vi "ExecutingCalibration.vi"(8 "error in (no error)":errorcluster, 10 "calibration_id":i32, 11 "ByteGSAPIBase in":refnum<class "ByteQXAPIBase.lvclass">) -> (0 "error out":errorcluster, 2 "calibration data":T1 {"controls"."umidita" format="%.1g"; "controls"."temperatura_c" format="%.1g"; "controls"."incertezza" format="%.1g"; "controls"."deviazione_standard" format="%.1g"; "controls"."mpe_min" format="%.1g"; "controls"."mpe_max" format="%.1g"; "controls"."riferimento_obiettivo" format="%.1g"}, 3 "ByteGSAPIBase out":refnum<class "ByteQXAPIBase.lvclass">)   [LabVIEW 2019, in "ByteQXWebAPI.lvlib" / "ByteQXAPIBase.lvclass"]
doc: "Obtain calibration measurements for the specified calibration Id"
uses:
  ByteQXAPIBase.lvclass
  BodyCalibrazioneMisure.ctl
  <vilib>/Bytelabs/ByteREST/ByteRESTClass/ByteRESTBase/HTTP/Status_Code.ctl
  ByteQXAPIBase.lvclass/ByteQXAPIBase.ctl
  <vilib>/Utility/error.llb/Error Cluster From Error Code.vi
  <vilib>/ErrorRing/Error Ring.xnode
  <vilib>/Bytelabs/ByteREST/ByteRESTClass/ByteRESTBase/RESTBase.lvclass
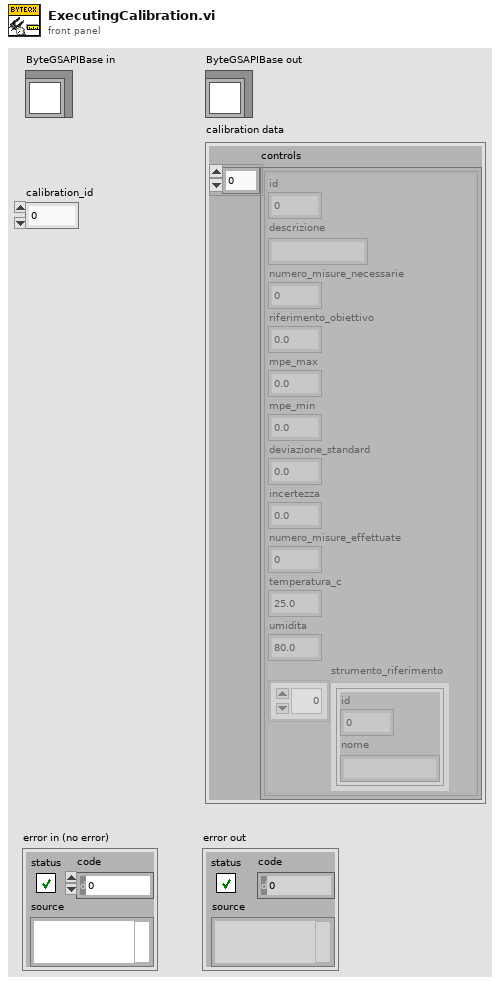
[diagram p1: front panel]
types:
  T1 = typedef "ByteQXWebAPI.lvlib/ByteQXAPIBase.lvclass/BodyCalibrazioneMisure.ctl" = cluster{"controls":cluster{"id":u16, "descrizione":string, "numero_misure_necessarie":u16, "riferimento_obiettivo":dbl, "mpe_max":dbl, "mpe_min":dbl, "deviazione_standard":dbl, "incertezza":dbl, "numero_misure_effettuate":u32, "temperatura_c":dbl, "umidita":dbl, "strumento_riferimento":cluster{"id":u16, "nome":string}[]}[]}
  T2 = typedef "ByteREST.lvlib/RESTBase.lvclass/Status_Code.ctl" = u16
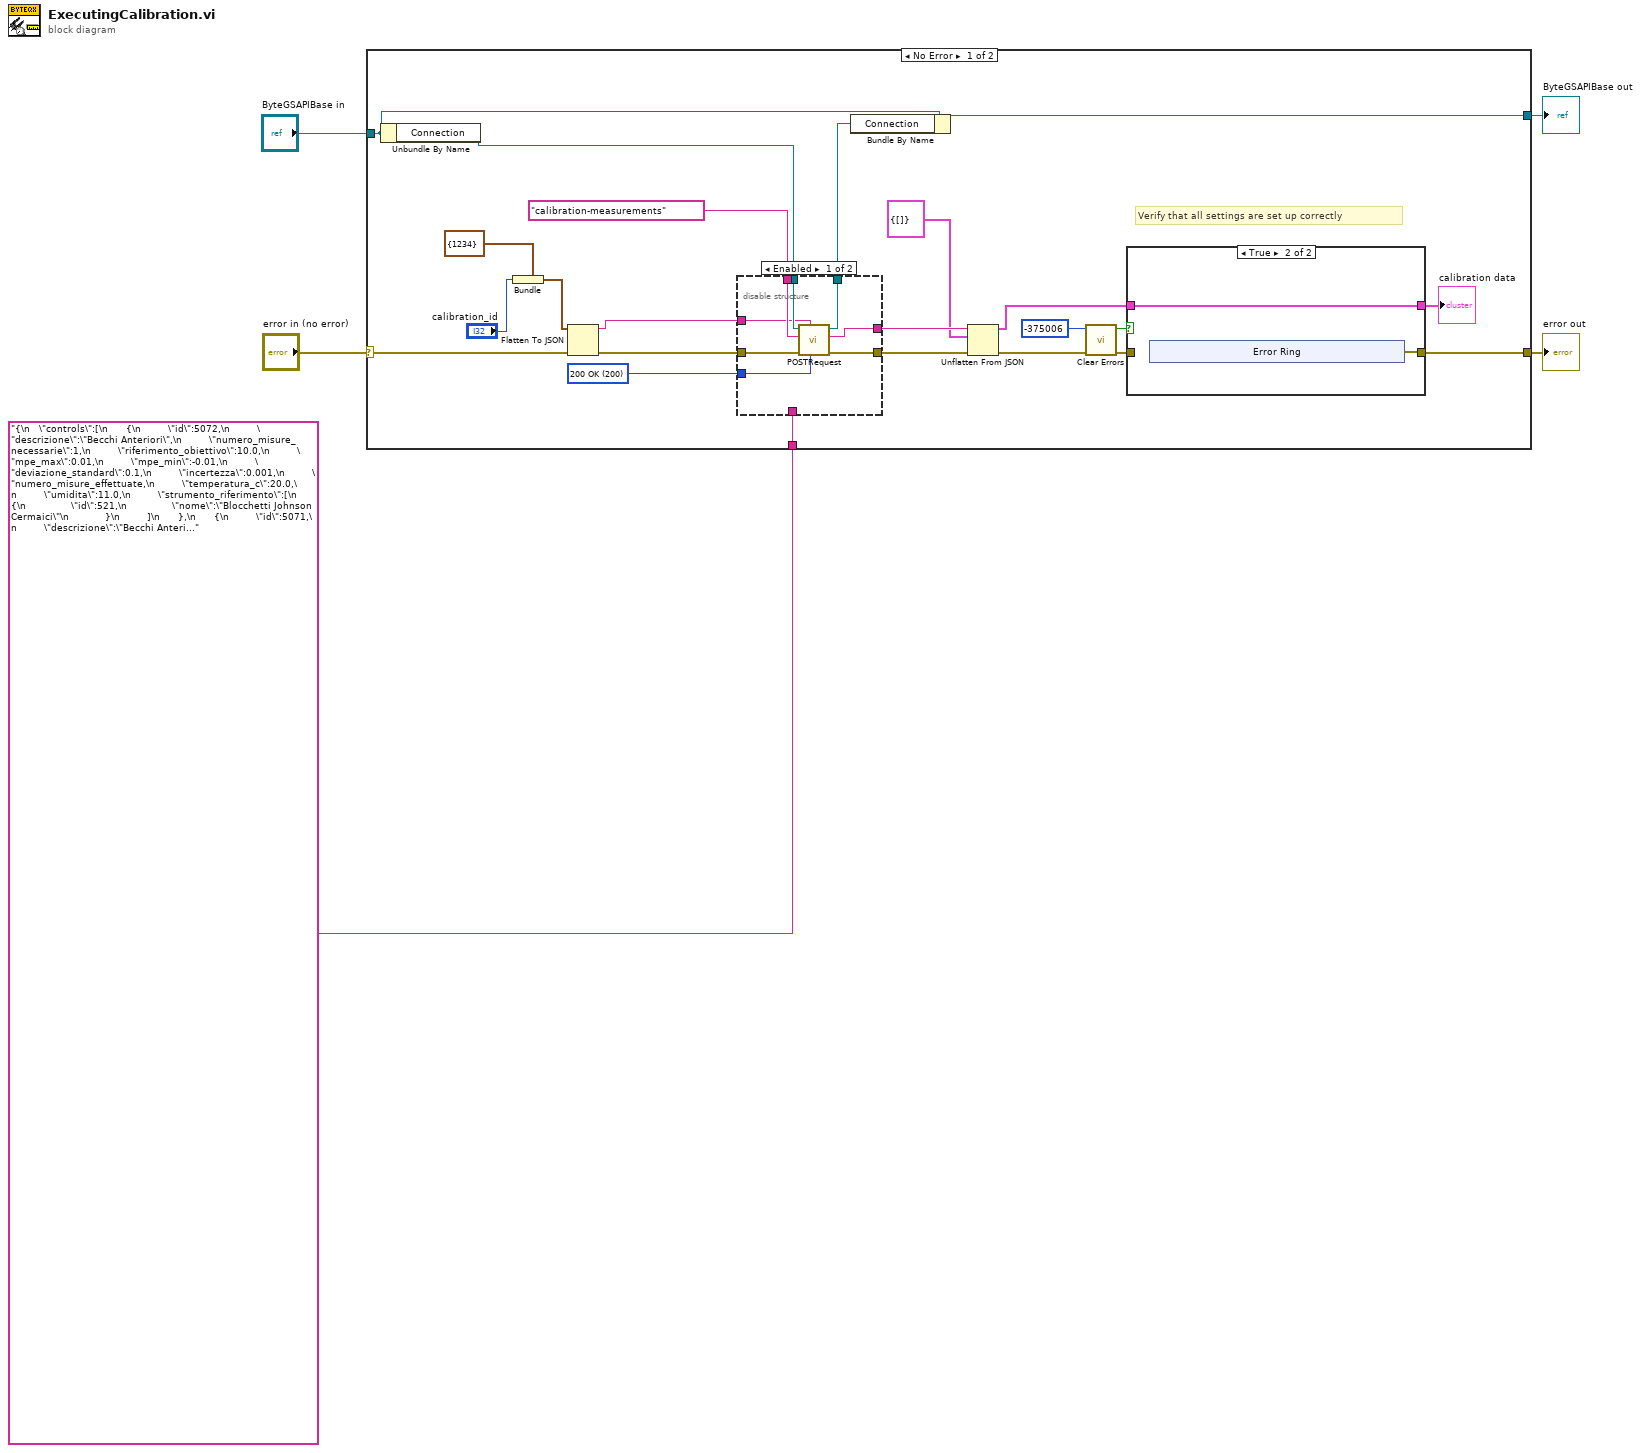
[diagram p0: block diagram]
diagram:
  n1 = case shown="No Error" "error in (no error)" {
    selector: "error in (no error)" -> [w23 w50]
    tunnel: [w9 w50] -> w4
    tunnel: [w26 w49] -> w2
    tunnel: "ByteGSAPIBase in" -> [w28 w49]
    tunnel: "{\n   \"controls\":[\n      {\n         \"id\":5072,\n         \"descrizione\":\"Becchi Anteriori\",\n         \"numero_misure_necessarie\":1,\n         \"riferimento_obiettivo\":10.0,\n         \"mpe_max\":0.01,\n         \"mpe_min\":-0.01,\n         \"deviazione_standard\":0.1,\n         \"incertezza\":0.001,\n         \"numero_misure_effettuate,\n         \"temperatura_c\":20.0,\n         \"umidita\":11.0,\n         \"strumento_riferimento\":[\n            {\n               \"id\":521,\n               \"nome\":\"Blocchetti Johnson Cermaici\"\n            }\n         ]\n      },\n      {\n         \"id\":5071,\n         \"descrizione\":\"Becchi Anteriori\",\n         \"numero_misure_necessarie\":1,\n         \"riferimento_obiettivo\":15.0,\n         \"mpe_max\":0.01,\n         \"mpe_min\":-0.01,\n         \"deviazione_standard\":0.1,\n         \"incertezza\":0.001,\n         \"numero_misure_effettuate,\n         \"temperatura_c\":18.0,\n         \"umidita\":10.0,\n         \"strumento_riferimento\":[\n            {\n               \"id\":521,\n               \"nome\":\"Blocchetti Johnson Cermaici\"\n            }\n         ]\n      },\n      {\n         \"id\":5070,\n         \"descrizione\":\"Profondità\",\n         \"numero_misure_necessarie\":1,\n         \"riferimento_obiettivo\":20.0,\n         \"mpe_max\":0.01,\n         \"mpe_min\":-0.01,\n         \"deviazione_standard\":0.1,\n         \"incertezza\":0.001,\n         \"temperatura_c\":18.0,\n         \"umidita\":10.0,\n         \"strumento_riferimento\":[\n            {\n               \"id\":3974,\n               \"nome\":\"Micrometro a 3 punte\"\n            }\n         ]\n      }\n   ]\n}" -> [w13 _]
    frame No Error {
      w20 = T2 200 items=["200 OK"=200, "201 Created"=201, "400 Bad Request"=400, "401 Unauthorized"=401, "403 Forbidden"=403, "404 Not Found"=404, "405 Method Not Allowed"=405, "406 Not Acceptable"=406, "500 Internal Server Error"=500] ("expected response")
      # "Verify that all settings are set up correctly"
      n2 = Unbundle By Name(w28) -> ("Connection"=w27:refnum<class "RESTBase.lvclass">)
      n3 = Bundle(cluster=cluster{"calibration_id":i32} {"calibration_id"=1234}, "calibration_id"="calibration_id") -> (w14:cluster{"calibration_id":i32})
      n4 = Flatten To JSON(anything=w14, error in (no error)=w23) -> (JSON string=w18:string, 11:w19:errorcluster)  [unwired: 1 in]
      n5 = disable-structure shown="Enabled" {
        disable-tunnel: w27 -> [w45 w46]
        disable-tunnel: [w44 w46] -> w25
        disable-tunnel: "calibration-measurements" ("Request") -> [w43 _]
        disable-tunnel: [w42 w48] -> w22
        disable-tunnel: [w41 w47] -> w21
        disable-tunnel: w20 -> [w40 _]
        disable-tunnel: w19 -> [w39 w47]
        disable-tunnel: w18 -> [w38 _]
        disable-tunnel: w13 -> [_ w48]
        frame Enabled {
          n6 = call-dynamic "POSTRequest.vi"("expected response"=w40, "Body in"=w38, "error in (no error)"=w39, "Request"=w43, "ByteRESTBase in"=w45) -> ("error out"=w41:errorcluster, "Body"=w42:string, "ByteRESTBase out"=w44:refnum<class "RESTBase.lvclass">)  [unwired: 3 in, 1 out]
        }
        frame Disabled {
        }
      }
      n7 = Bundle By Name(cluster=w28, "Connection"=w25) -> (w26:refnum<class "ByteQXAPIBase.lvclass">)
      n8 = Unflatten From JSON(JSON string=w22, type and defaults=T1 {"controls"=[]} ("Cluster 2"), error in (no error)=w21) -> (value=w7:T1, error out=w11:errorcluster)  [unwired: 4 in]
      n9 = call <vilib>:"Clear Errors.vi"("error in (no error)"=w11, "specific error code to clear (0: all)"=-375006 ("error code (no error:0)")) -> ("error out"=w10:errorcluster, "specific error cleared?"=w8:bool)  [unwired: 4 in]
      n10 = case shown="True" w8 {
        tunnel: w10 -> [w30 _]
        tunnel: [w30 w31] -> w9
        tunnel: w7 -> [w29 w32]
        tunnel: [w29 w32] -> w6
        frame False {
        }
        frame True {
          n11 = xnode "Error Ring"() -> ("error out"=w31:errorcluster)
        }
      }
      "calibration data" <- w6
    }
    frame Error {
    }
  }
  "error out" <- w4
  "ByteGSAPIBase out" <- w2
